vi "Actor Core.vi"(8 "error in":errorcluster, 11 "hydraharp_panel in":refnum<class "picoharp_panel.lvclass">) -> (0 "error out":errorcluster, 3 "Actor out":refnum<class "Actor.lvclass">)   [LabVIEW 2015, in "picoharp_panel.lvclass"]
doc: "(<B>Filename</B>: Actor Framework.lvlib:Actor.lvclass:Actor Core.vi)\n\nReceives messages to the actor, reacts to them, and initiates any error handling that may shut the actor down.\n\nDescendant classes may override this VI to append parallel tasks for the actor to complete while it handles messages. Overrides use the Call Parent Method node."
uses:
  picoharp_panel.lvclass
  <vilib>/ActorFramework/Actor/Actor.lvclass
  Hydraharp/hydraharp_panel/hpanel_hydraharp_settings.ctl
  Hydraharp/hydraharp_panel/hpanel_sync_settings.ctl
  Hydraharp/hydraharp_panel/hpanel_sync_div.ctl
  Hydraharp/hydraharp_panel/hpanel_channel_settings.ctl
  Hydraharp/hydraharp_panel/hpanel_acq_modes.ctl
  Hydraharp/hydraharp_panel/hpanel_hydrharp_tasks.ctl
  Hydraharp/hydraharp/hydraharp_correlation_lag_settings.ctl
  Hydraharp/hydraharp/hydraharp_time_decades.ctl
  Hydraharp/hydraharp_panel/hpanel_control_references.ctl
  UI/panel_class/panel.lvclass/panel.ctl
  <vilib>/ActorFramework/Actor/Actor.lvclass/Actor.ctl
  <vilib>/ActorFramework/Message Enqueuer/Message Enqueuer.lvclass/Message Enqueuer.ctl
  picoharp_panel.lvclass/picoharp_panel.ctl
  picoharp_panel Messages/ppanel_connect_to_hydraharp Msg/ppanel_connect_to_hydraharp Msg.lvclass/ppanel_connect_to_hydraharp Msg.ctl
  record_type.ctl
  Hydraharp/hydraharp/hydraharp_action_on_records.ctl
  picoharp_panel Messages/ppanel_stream_TTTR Msg/ppanel_stream_TTTR Msg.lvclass/ppanel_stream_TTTR Msg.ctl
  Hydraharp/hydraharp_panel/hpanel_correlation_settings.ctl
  picoharp_panel Messages/ppanel_change_hydraharp_settings Msg/ppanel_change_hydraharp_settings Msg.lvclass/ppanel_change_hydraharp_settings Msg.ctl
  <vilib>/ActorFramework/Message Enqueuer/Init from Existing Queue.vi
  <vilib>/ActorFramework/Message Enqueuer/Enqueue.vi
  <vilib>/ActorFramework/Message Priority Queue/Priority Enqueue.vi
  <vilib>/ActorFramework/Message Enqueuer/Message Enqueuer.lvclass
  picoharp_panel Messages/ppanel_disconnect_from_hydraharp Msg/ppanel_disconnect_from_hydraharp Msg.lvclass
  picoharp_panel Messages/ppanel_connect_to_hydraharp Msg/ppanel_connect_to_hydraharp Msg.lvclass
  picoharp_panel Messages/ppanel_get_current_count_rates Msg/ppanel_get_current_count_rates Msg.lvclass
  picoharp_panel Messages/ppanel_stream_TTTR Msg/ppanel_stream_TTTR Msg.lvclass
  picoharp_panel Messages/ppanel_change_hydraharp_settings Msg/ppanel_change_hydraharp_settings Msg.lvclass
  UI/panel_class/panel.lvclass
panel:
  in  "stop_task":bool
  in  "do_task":bool
  in  "Task":T1
  in  "chart_channels":bool
  in  "Mode":T2=2 items=["T2"=2, "T3"=3]
  out "Status":string
  in  "connect_hydraharp":bool
  in  "hydra_tab":enum32{"Basic Settings", "Advanced"}(tab)
  in  "Hydraharp Settings":T3={"Sync Settings"={"snc_count"=0, "snc_level"=50, "snc_ZeroX"=10, "snc_offs"=0, "sync_div"=enum."1"}, "CH 1"={"ch_counts"=0, "ch_level"=270, "ch_ZeroX"=10, "ch_offs"=0}, "CH 2"={"ch_counts"=0, "ch_level"=680, "ch_ZeroX"=10, "ch_offs"=0}, "CH 3"={"ch_counts"=0, "ch_level"=50, "ch_ZeroX"=10, "ch_offs"=0}, "CH 4"={"ch_counts"=0, "ch_level"=50, "ch_ZeroX"=10, "ch_offs"=0}, "binning"=1, "CH 5"={"ch_counts"=0, "ch_level"=0, "ch_ZeroX"=0, "ch_offs"=0}, "CH 6"={"ch_counts"=0, "ch_level"=0, "ch_ZeroX"=0, "ch_offs"=0}, "CH 7"={"ch_counts"=0, "ch_level"=0, "ch_ZeroX"=0, "ch_offs"=0}, "CH 8"={"ch_counts"=0, "ch_level"=0, "ch_ZeroX"=0, "ch_offs"=0}} {"CH 8"."ch_offs" min=-99999 max=99999 step=1; "CH 8"."ch_ZeroX" min=0 max=20 step=1; "CH 8"."ch_level" min=0 max=800 step=1; "CH 7"."ch_offs" min=-99999 max=99999 step=1; "CH 7"."ch_ZeroX" min=0 max=20 step=1; "CH 7"."ch_level" min=0 max=800 step=1; "CH 6"."ch_offs" min=-99999 max=99999 step=1; "CH 6"."ch_ZeroX" min=0 max=20 step=1; "CH 6"."ch_level" min=0 max=800 step=1; "CH 5"."ch_offs" min=-99999 max=99999 step=1; "CH 5"."ch_ZeroX" min=0 max=20 step=1; "CH 5"."ch_level" min=0 max=800 step=1; "binning" min=0 max=10 step=1; "CH 4"."ch_offs" min=-99999 max=99999 step=1; "CH 4"."ch_ZeroX" min=0 max=20 step=1; "CH 4"."ch_level" min=0 max=800 step=1; "CH 3"."ch_offs" min=-99999 max=99999 step=1; "CH 3"."ch_ZeroX" min=0 max=20 step=1; "CH 3"."ch_level" min=0 max=800 step=1; "CH 2"."ch_offs" min=-99999 max=99999 step=1; "CH 2"."ch_ZeroX" min=0 max=20 step=1; "CH 2"."ch_level" min=0 max=800 step=1; "CH 1"."ch_offs" min=-99999 max=99999 step=1; "CH 1"."ch_ZeroX" min=0 max=20 step=1; "CH 1"."ch_level" min=0 max=800 step=1; "Sync Settings"."snc_offs" min=-99999 max=99999 step=1; "Sync Settings"."snc_ZeroX" min=0 max=20 step=1; "Sync Settings"."snc_level" min=0 max=800 step=10}
  in  "acq_time (s)":u32=100
  in  "Stream Path":path
  in  "Ch2":u8 max=16
  in  "Ch1":u8 max=16
  in  "Lag Settings":T7={"time_start"=1000000, "time_end"=100000000000, "coarseness"=4} {"time_start" items=["1 ps"=1, "10 ps"=10, "100 ps"=100, "1 ns"=1000, "10 ns"=10000, "100 ns"=100000, "1 us"=1000000, "10 us"=10000000, "100 us"=100000000, "1 ms"=1000000000, "10 ms"=10000000000, "100 ms"=100000000000, "1 s"=1000000000000, "10 s"=10000000000000, "100 s"=100000000000000]; "time_end" items=["1 ps"=1, "10 ps"=10, "100 ps"=100, "1 ns"=1000, "10 ns"=10000, "100 ns"=100000, "1 us"=1000000, "10 us"=10000000, "100 us"=100000000, "1 ms"=1000000000, "10 ms"=10000000000, "100 ms"=100000000000, "1 s"=1000000000000, "10 s"=10000000000000, "100 s"=100000000000000]}
  in  "Save Records?":bool
  # "PicoHarp"
  # "CH 0"
  # "CH 1"
  # "Stream Settings"
  # "Correlation Settings"
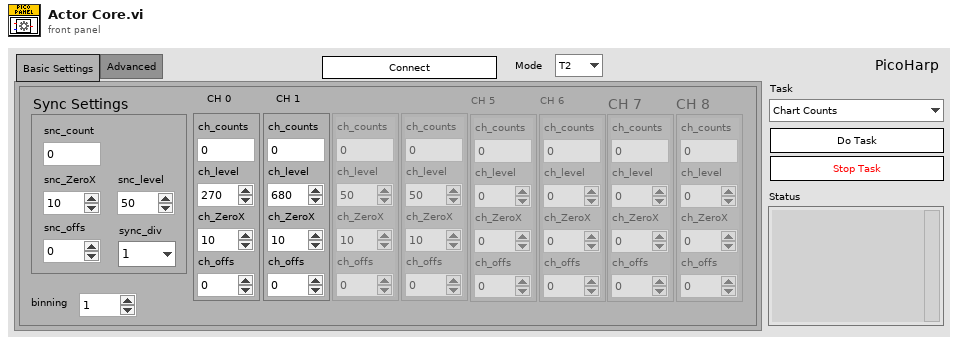
[diagram p1: front panel]
types:
  T1 = typedef "hpanel_hydrharp_tasks.ctl" = enum16{"Chart Counts", "Stream to File", "Plot Correlation"}
  T2 = typedef "hpanel_acq_modes.ctl" = u16
  T3 = typedef "hpanel_hydraharp_settings.ctl" = cluster{"Sync Settings":T4, "CH 1":T6, "CH 2":T6, "CH 3":T6, "CH 4":T6, "binning":i32, "CH 5":T6, "CH 6":T6, "CH 7":T6, "CH 8":T6}
  T4 = typedef "hpanel_sync_settings.ctl" = cluster{"snc_count":i32, "snc_level":i32, "snc_ZeroX":i32, "snc_offs":i32, "sync_div":T5}
  T5 = typedef "hpanel_sync_div.ctl" = enum16{"1", "2", "4", "8"}
  T6 = typedef "hpanel_channel_settings.ctl" = cluster{"ch_counts":i32, "ch_level":i32, "ch_ZeroX":i32, "ch_offs":i32}
  T7 = typedef "hydraharp_correlation_lag_settings.ctl" = cluster{"time_start":T8, "time_end":T8, "coarseness":i64}
  T8 = typedef "hydraharp_time_decades.ctl" = i64
  T9 = typedef "hpanel_control_references.ctl" = cluster{"Status":refnum<vi>, "snc_count":refnum<vi>, "ch1_counts":refnum<vi>, "ch2_counts":refnum<vi>, "ch3_counts":refnum<vi>, "ch4_counts":refnum<vi>, "ch5_counts":refnum<vi>, "ch6_counts":refnum<vi>, "ch7_counts":refnum<vi>, "ch8_counts":refnum<vi>}
  T10 = typedef "hpanel_user_events.ctl" = cluster{"message_panel":refnum<event-registration>, "stop_fifo_stream":refnum<event-registration>, "harp_status":refnum<event-registration>}
  T11 = cluster{"message_panel":refnum<event-registration>, "stop_ui_ref":refnum<event-registration>, "harp_status":refnum<event-registration>}
  T12 = typedef "record_type.ctl" = enum16{"Raw Stream", "Processed Records (hdf5)"}
  T13 = enum8{"Enabled", "Disabled", "Disabled and Grayed Out"}
  T14 = typedef "hydraharp_action_on_records.ctl" = enum16{"stream_to_file", "correlate", "stream to file and correlate"}
  T15 = typedef "hpanel_correlation_settings.ctl" = cluster{"Lag Settings":T7, "Ch1":u8, "Ch2":u8}
  T16 = typedef "ui_user_events.ctl" = cluster{"update_xy_graph":refnum<user-event>, "update_graph":refnum<user-event>, "update_chart":refnum<user-event>, "update_map":refnum<user-event>, "event_loop_stop":refnum<user-event>, "keep_map":refnum<user-event>}
  T17 = typedef "hydrharp_tasks.ctl" = enum16{"Chart Counts", "Stream to File", "Plot Correlation"}
  T18 = typedef "messages_to_panel_from_actor_loop.ctl" = enum16{"reenable_tasks"}
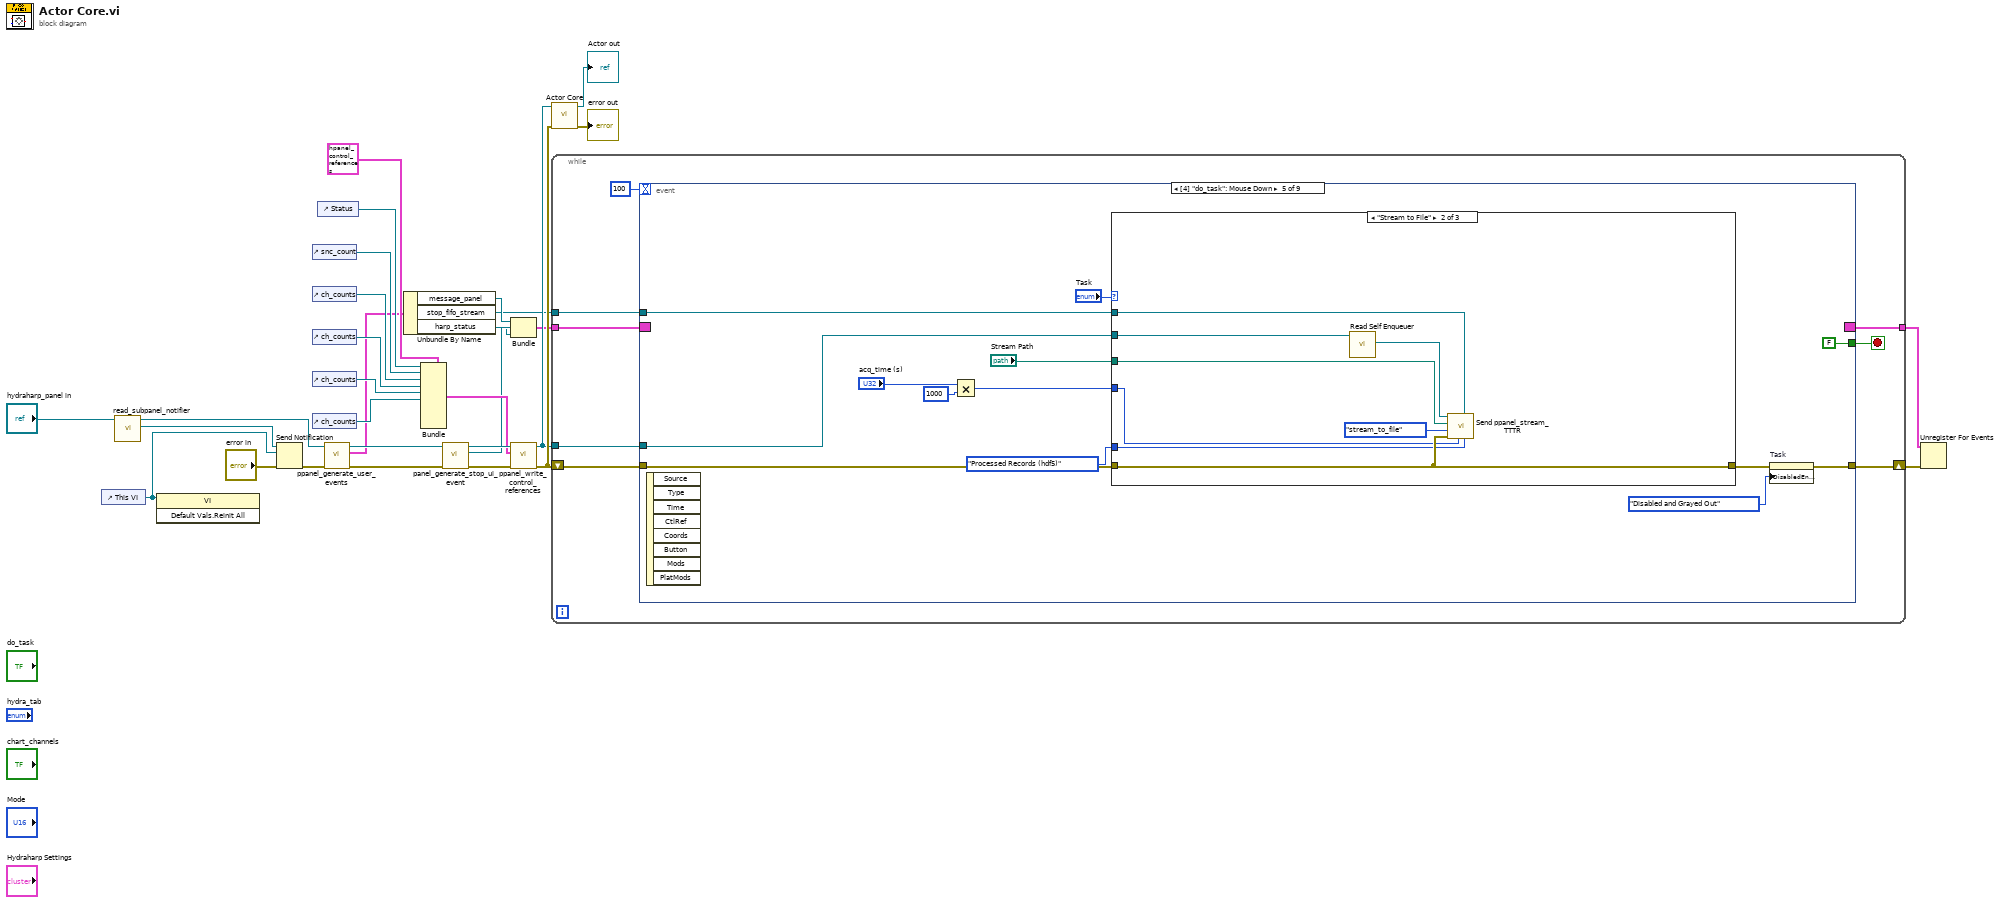
[diagram p0: block diagram]
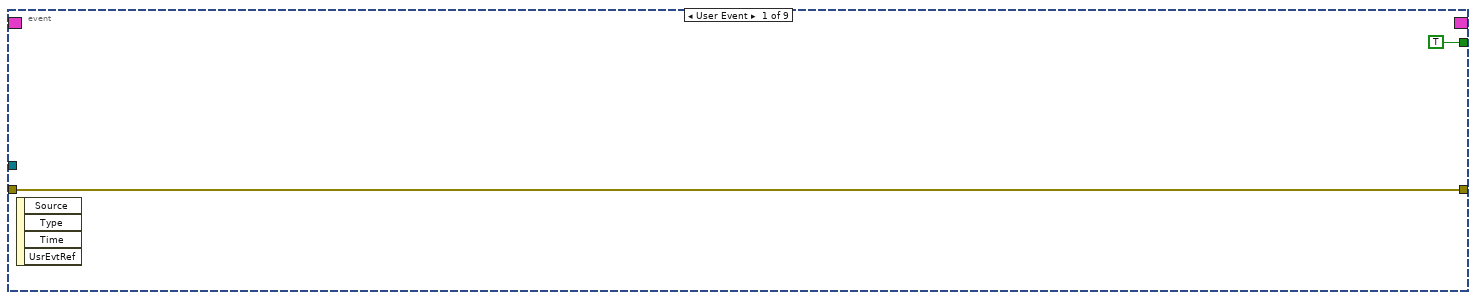
[diagram p2: hidden frame]
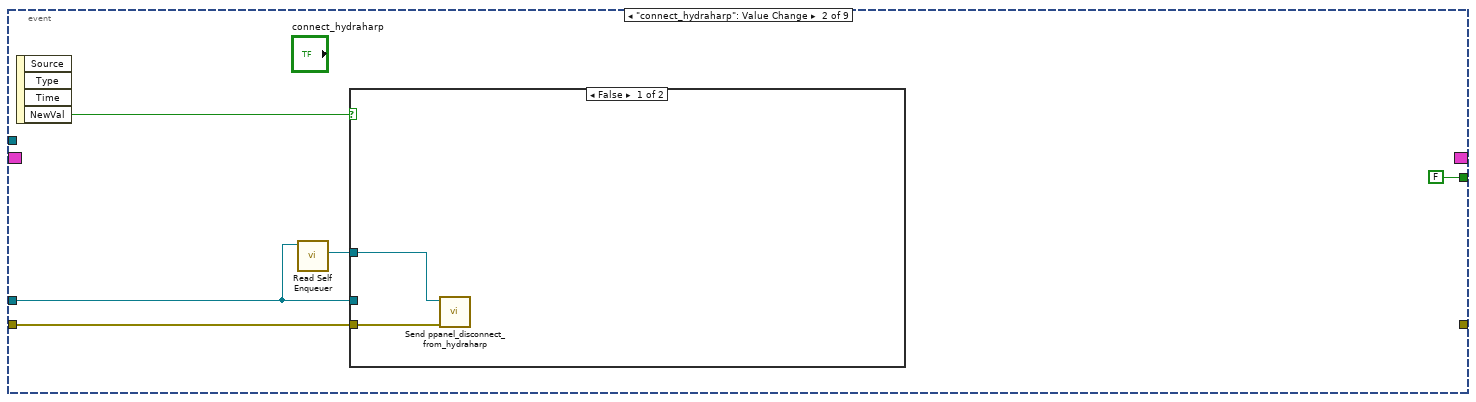
[diagram p3: hidden frame]
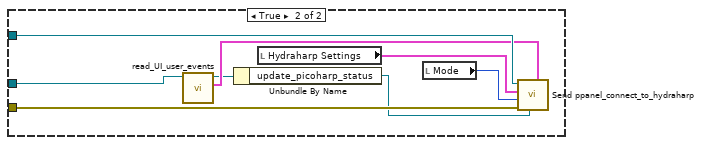
[diagram p4: hidden frame]
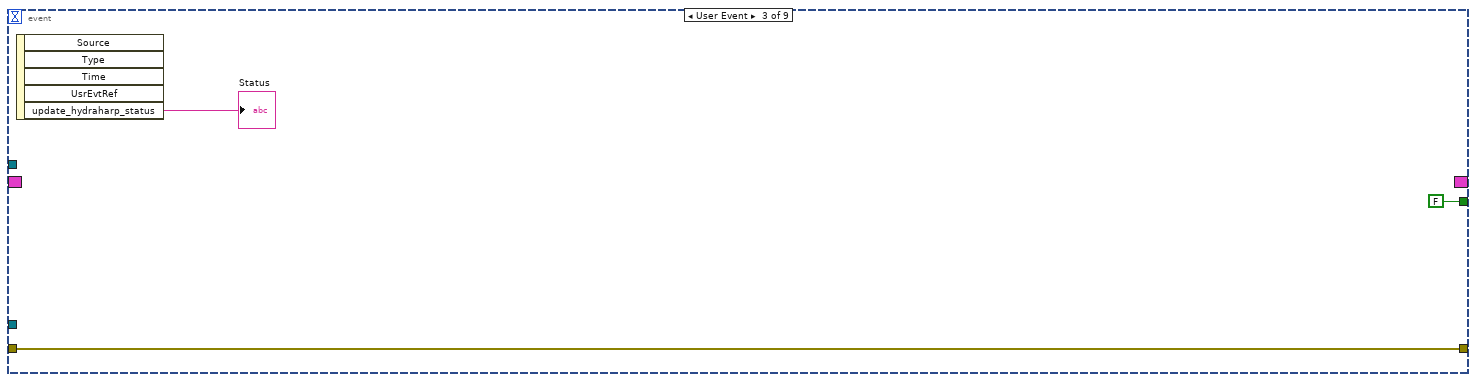
[diagram p5: hidden frame]
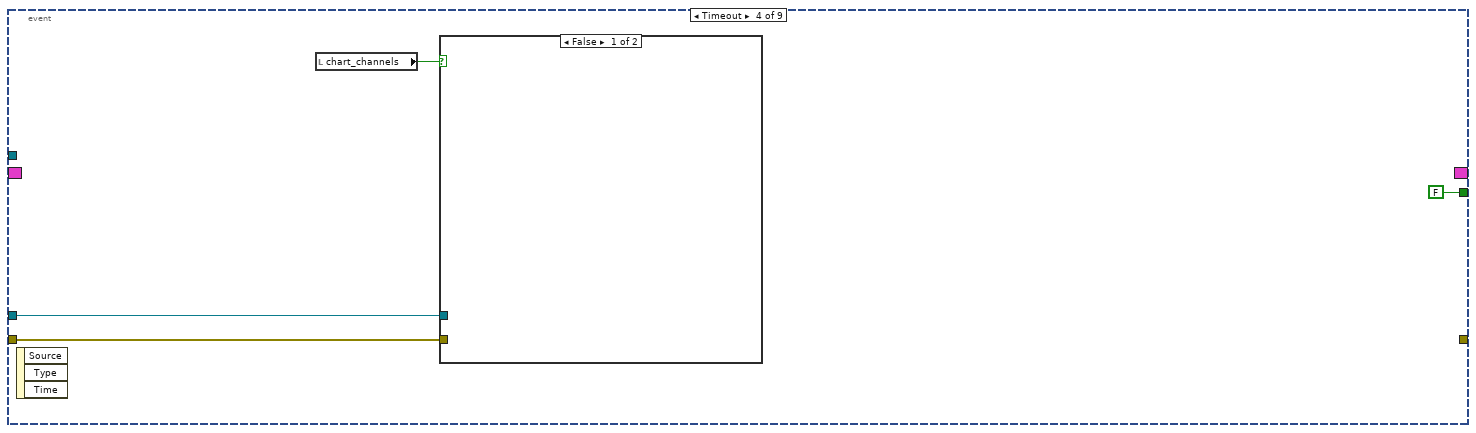
[diagram p6: hidden frame]
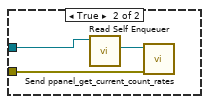
[diagram p7: hidden frame]
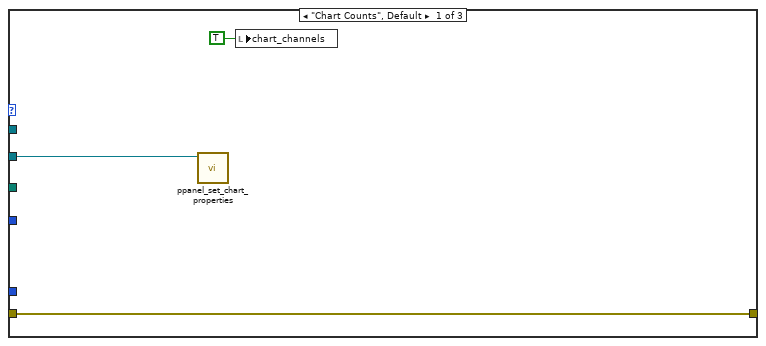
[diagram p8: hidden frame]
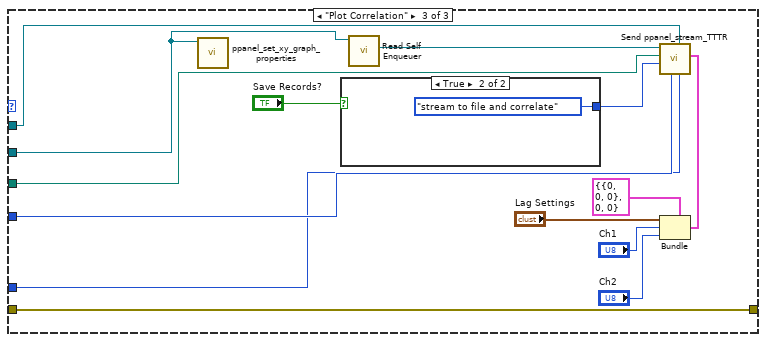
[diagram p9: hidden frame]
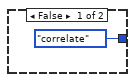
[diagram p10: hidden frame]
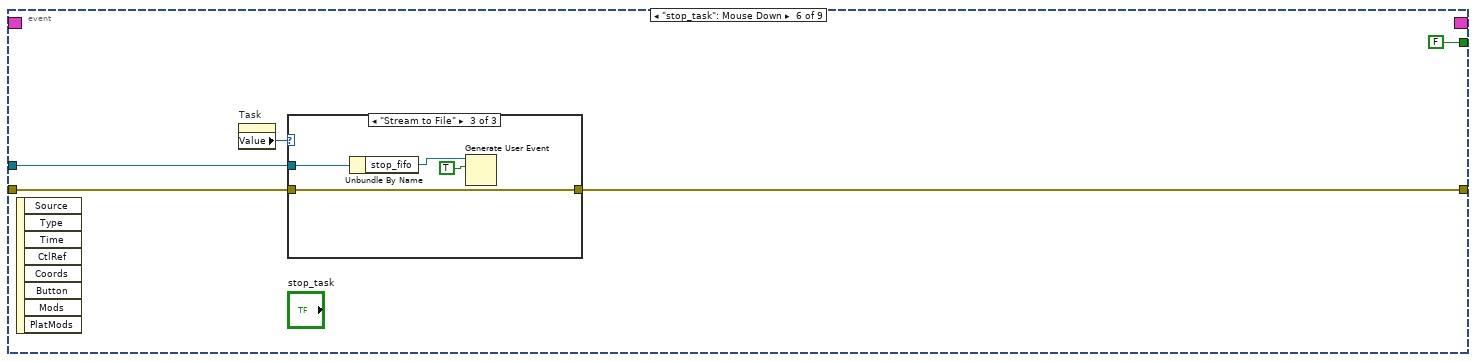
[diagram p11: hidden frame]
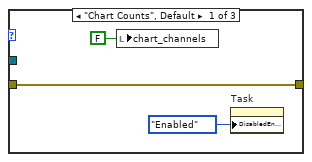
[diagram p12: hidden frame]
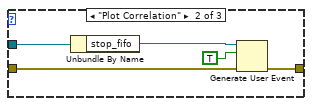
[diagram p13: hidden frame]
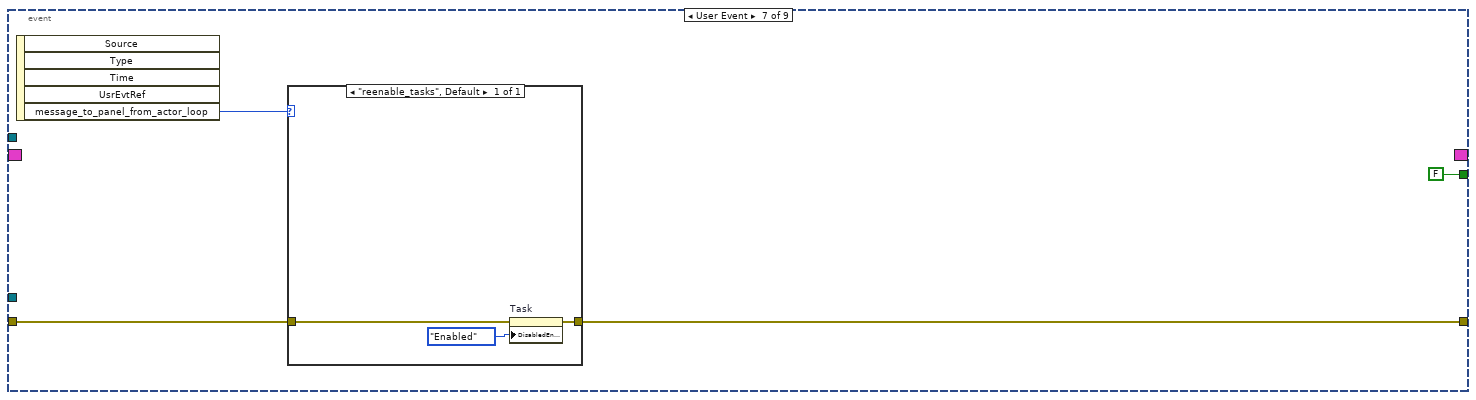
[diagram p14: hidden frame]
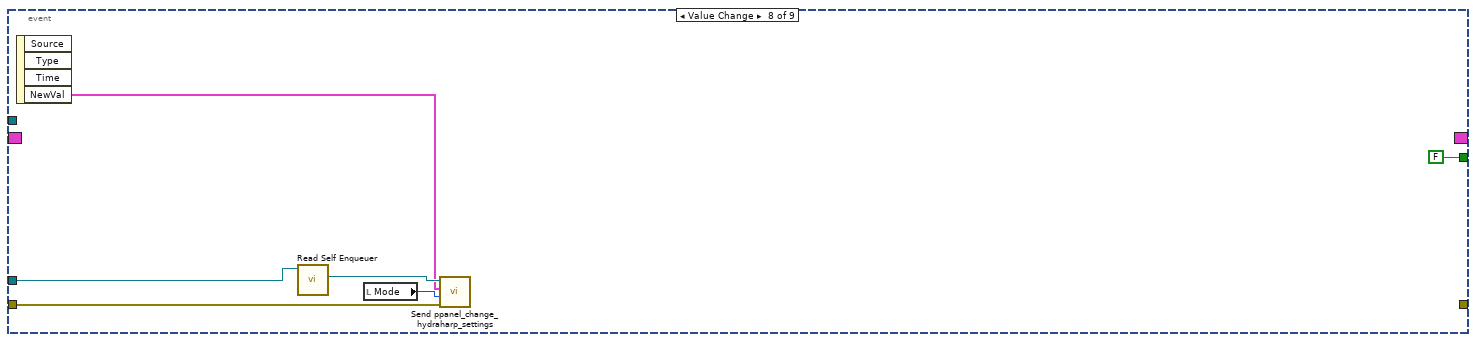
[diagram p15: hidden frame]
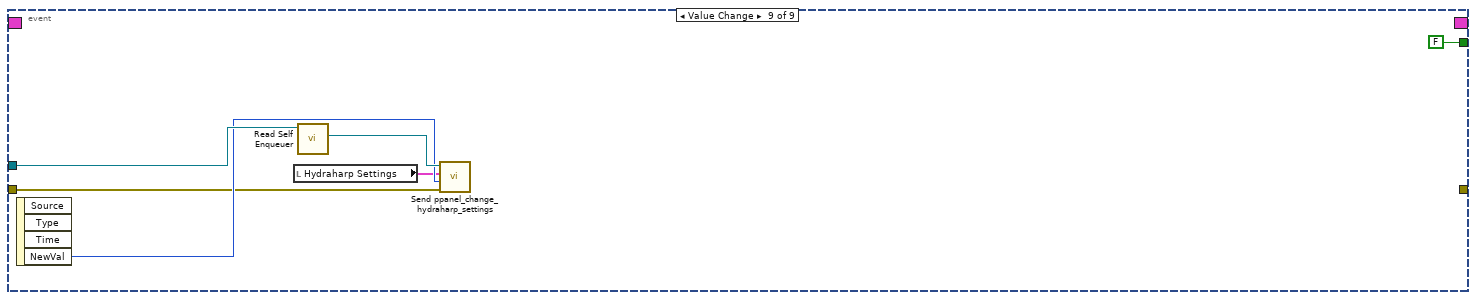
[diagram p16: hidden frame]
diagram:
  n1 = control-ref of="This VI"() -> (w13:refnum<vi>)
  n2 = call "read_subpanel_notifier.vi"("panel in"="hydraharp_panel in") -> ("subpanel_notifier"=w1:refnum<notifier>, "panel out"=w2:refnum<class "picoharp_panel.lvclass">)  [unwired: 8 in, 1 out]
  n3 = invoke class="VI" method="Default Vals.Reinit All"(reference=w13) -> ()  [unwired: 2 in, 3 out]
  n4 = Send Notification(notification=w13, notifier=w1, error in (no error)="error in") -> (error out=w12:errorcluster)  [unwired: 1 out]
  n5 = control-ref of="snc_count"() -> (w24:refnum<vi>)
  n6 = control-ref of="ch_counts"() -> (w23:refnum<vi>)
  n7 = control-ref of="ch_counts"() -> (w22:refnum<vi>)
  n8 = control-ref of="ch_counts"() -> (w21:refnum<vi>)
  n9 = control-ref of="ch_counts"() -> (w20:refnum<vi>)
  n10 = control-ref of="Status"() -> (w25:refnum<vi>)
  n11 = call "ppanel_generate_user_events.vi"("error in (no error)"=w12, "picoharp_panel in"=w2) -> ("error out"=w11:errorcluster, "events"=w8:T10, "hydraharp_panel out"=w10:refnum<class "picoharp_panel.lvclass">)  [unwired: 7 in]
  n12 = Unbundle By Name(w8) -> ("message_panel"=w7:refnum<event-registration>, "stop_fifo_stream"=w5:refnum<event-registration>, "harp_status"=w4:refnum<event-registration>)
  n13 = Bundle(cluster=T9 {"Status"=refnum, "snc_count"=refnum, "ch1_counts"=refnum, "ch2_counts"=refnum, "ch3_counts"=refnum, "ch4_counts"=refnum, "ch5_counts"=refnum, "ch6_counts"=refnum, "ch7_counts"=refnum, "ch8_counts"=refnum} ("output cluster"), "Status"=w25, "snc_count"=w24, "ch1_counts"=w23, "ch2_counts"=w22, "ch3_counts"=w21, "ch4_counts"=w20) -> (w15:T9)  [unwired: 4 in]
  n14 = call "panel_generate_stop_ui_event.vi"("error in (no error)"=w11, "panel in"=w10) -> ("error out"=w17:errorcluster, "stop_ui_ref"=w9:refnum<event-registration>, "panel out"=w18:refnum<class "picoharp_panel.lvclass">)  [unwired: 7 in]
  n15 = Bundle("message_panel"=w7, "stop_ui_ref"=w9, "harp_status"=w4) -> (w6:T11)  [unwired: 1 in]
  n16 = call "ppanel_write_control_references.vi"("error in (no error)"=w17, "references"=w15, "hydraharp_panel in"=w18) -> ("error out"=w16:errorcluster, "hydraharp_panel out"=w14:refnum<class "picoharp_panel.lvclass">)  [unwired: 7 in]
  n17 = call-parent "Actor Core.vi"("error in"=w16, "Actor in"=w14) -> ("error out"=→"error out":errorcluster, "Actor out"=→"Actor out":refnum<class "Actor.lvclass">)  [unwired: 8 in]
  n18 = while {
    tunnel: [w38] -> w27
    shift-right: [w35] -> w26
    shift-left: w16 -> [w36]
    tunnel: w14 -> [w34]
    tunnel: w6 -> [w32]
    tunnel: w5 -> [w31]
    stop <- w37 stop-if-true
    n19 = event shown="[4] \"do_task\": Mouse Down" {
      selector: w32 -> [_ _ _ _ _ _ _ _ _]
      dyn-events: [_ _ _ _ _ _ _ _ _] -> w38
      timeout: 100 -> [_ _ _ _ _ _ _ _ _]
      tunnel: [TRUE FALSE FALSE FALSE FALSE FALSE FALSE FALSE FALSE] -> w37
      tunnel: w36 -> [w39 w45 w56 w60 w76 w109 w124 w130 w137]
      tunnel: [w39 _ w56 _ w74 w106 w123 _ _] -> w35
      tunnel: w34 -> [_ w41 _ w61 w72 w107 _ w135 w141]
      tunnel: w31 -> [_ _ _ _ w71 _ _ _ _]
      event User Event {
        n20 = event-data() -> ()  [unwired: 1 in, 4 out]
      }
      event "connect_hydraharp": Value Change {
        n21 = event-data() -> ("NewVal"=w43:bool)  [unwired: 1 in, 3 out]
        n22 = call <vilib>:"Read Self Enqueuer.vi"("Actor"=w41) -> ("Self Enqueuer"=w44:refnum<class "Message Enqueuer.lvclass">)  [unwired: 10 in]
        n23 = case shown="False" w43 {
          tunnel: w45 -> [w46 w55]
          tunnel: w44 -> [w47 w54]
          tunnel: w41 -> [_ w50]
          frame False {
            n24 = call "Send ppanel_disconnect_from_hydraharp.vi"("error in (no error)"=w46, "Message Enqueuer"=w47) -> ()  [unwired: 8 in, 2 out]
          }
          frame True {
            n25 = call "read_UI_user_events.vi"("panel in"=w50) -> ("ui_user_events"=w49:T16, "panel out"=w48:refnum<class "picoharp_panel.lvclass">)  [unwired: 8 in, 1 out]
            n26 = Unbundle By Name(w48) -> ("update_picoharp_status"=w51:refnum<user-event>)
            n27 = local read "Hydraharp Settings"() -> (w53:T3)
            n28 = local read "Mode"() -> (w52:T2)
            n29 = call "Send ppanel_connect_to_hydraharp.vi"("ui_events"=w49, "update_hydraharp_status"=w51, "error in (no error)"=w55, "Mode"=w52, "Hydraharp Settings"=w53, "Message Enqueuer"=w54) -> ()  [unwired: 4 in, 2 out]
          }
        }
      }
      event User Event {
        n30 = event-data() -> ("update_hydraharp_status"=→"Status":string)  [unwired: 1 in, 4 out]
      }
      event Timeout {
        n31 = event-data() -> ()  [unwired: 1 in, 3 out]
        n32 = local read "chart_channels"() -> (w59:bool)
        n33 = case shown="False" w59 {
          tunnel: w61 -> [_ w65]
          tunnel: w60 -> [_ w63]
          frame False {
          }
          frame True {
            n34 = call <vilib>:"Read Self Enqueuer.vi"("Actor"=w65) -> ("Self Enqueuer"=w64:refnum<class "Message Enqueuer.lvclass">)  [unwired: 10 in]
            n35 = call "Send ppanel_get_current_count_rates.vi"("error in (no error)"=w63, "Message Enqueuer"=w64) -> ()  [unwired: 8 in, 2 out]
          }
        }
      }
      event "do_task": Mouse Down {
        n36 = event-data() -> ()  [unwired: 1 in, 8 out]
        n37 = Multiply(x="acq_time (s)", y=u32 1000) -> (x*y=w67:u32)
        n38 = case shown="\"Stream to File\"" "Task" {
          tunnel: w76 -> [w81 w89 w94]
          tunnel: [w81 w89 w94] -> w75
          tunnel: w72 -> [w79 w83 w92]
          tunnel: w71 -> [_ w86 w91]
          tunnel: "Stream Path" -> [_ w85 w97]
          tunnel: record_type."Processed Records (hdf5)" ("Record Type") -> [_ w82 w90]
          tunnel: w67 -> [_ w84 w96]
          frame "Chart Counts", Default {
            n39 = call "ppanel_set_chart_properties.vi"("hydraharp_panel in"=w79) -> ()  [unwired: 11 in]
            n40 = local write "chart_channels"(TRUE ("chart_channels")) -> ()
          }
          frame "Stream to File" {
            n41 = call <vilib>:"Read Self Enqueuer.vi"("Actor"=w83) -> ("Self Enqueuer"=w88:refnum<class "Message Enqueuer.lvclass">)  [unwired: 10 in]
            n42 = call "Send ppanel_stream_TTTR.vi"("Record Type"=w82, "stop_fifo_event"=w86, "acq_time"=w84, "error in (no error)"=w89, "action_for_records"=hydraharp_action_on_records."stream_to_file", "fifo_stream_path"=w85, "Message Enqueuer"=w88) -> ()  [unwired: 3 in, 2 out]
          }
          frame "Plot Correlation" {
            n43 = call "ppanel_set_xy_graph_properties.vi"("hydraharp_panel in"=w92) -> ()  [unwired: 11 in]
            n44 = case shown="True" "Save Records?" {
              tunnel: [hydraharp_action_on_records."correlate" ("action_for_records") hydraharp_action_on_records."stream to file and correlate" ("action_for_records")] -> w95
              frame False {
              }
              frame True {
              }
            }
            n45 = call <vilib>:"Read Self Enqueuer.vi"("Actor"=w92) -> ("Self Enqueuer"=w98:refnum<class "Message Enqueuer.lvclass">)  [unwired: 10 in]
            n46 = Bundle(cluster=T15 {"Lag Settings"={"time_start"=0, "time_end"=0, "coarseness"=0}, "Ch1"=0, "Ch2"=0} ("output cluster"), "Lag Settings"="Lag Settings", "Ch1"="Ch1", "Ch2"="Ch2") -> (w99:T15)
            n47 = call "Send ppanel_stream_TTTR.vi"("Correlation_settings"=w99, "Record Type"=w90, "stop_fifo_event"=w91, "acq_time"=w96, "action_for_records"=w95, "fifo_stream_path"=w97, "Message Enqueuer"=w98) -> ()  [unwired: 3 in, 2 out]
          }
        }
        n48 = property on="Task" class="Enum (strict)"(error in=w75, "DisabledEnum"=T13."Disabled and Grayed Out" ("Disabled")) -> (error out=w74:errorcluster)  [unwired: 1 in, 1 out]
      }
      event "stop_task": Mouse Down {
        n49 = event-data() -> ()  [unwired: 1 in, 8 out]
        n50 = property on="Task" class="Enum (strict)"() -> ("Value"=w110:T17)  [unwired: 2 in, 2 out]
        n51 = case shown="\"Stream to File\"" w110 {
          tunnel: w109 -> [w112 w115 w121]
          tunnel: [w112 w114 w121] -> w106
          tunnel: w107 -> [_ w116 w120]
          frame "Chart Counts", Default {
            n52 = local write "chart_channels"(FALSE ("chart_channels")) -> ()
            n53 = property on="Task" class="Enum (strict)"("DisabledEnum"=T13."Enabled" ("Disabled")) -> ()  [unwired: 2 in, 2 out]
          }
          frame "Plot Correlation" {
            n54 = Unbundle By Name(w116) -> ("stop_fifo"=w117:refnum<user-event>)
            n55 = Generate User Event(user event=w117, event data cluster=TRUE ("event data"), error in=w115) -> (error out=w114:errorcluster)  [unwired: 1 in, 1 out]
          }
          frame "Stream to File" {
            n56 = Unbundle By Name(w120) -> ("stop_fifo"=w119:refnum<user-event>)
            n57 = Generate User Event(user event=w119, event data cluster=TRUE ("event data")) -> ()  [unwired: 2 in, 2 out]
          }
        }
      }
      event User Event {
        n58 = event-data() -> ("message_to_panel_from_actor_loop"=w126:T18)  [unwired: 1 in, 4 out]
        n59 = case shown="\"reenable_tasks\", Default" w126 {
          tunnel: w124 -> [w128]
          tunnel: [w127] -> w123
          frame "reenable_tasks", Default {
            n60 = property on="Task" class="Enum (strict)"(error in=w128, "DisabledEnum"=T13."Enabled" ("Disabled")) -> (error out=w127:errorcluster)  [unwired: 1 in, 1 out]
          }
        }
      }
      event Value Change {
        n61 = event-data() -> ("NewVal"=w133:T3)  [unwired: 1 in, 3 out]
        n62 = call <vilib>:"Read Self Enqueuer.vi"("Actor"=w135) -> ("Self Enqueuer"=w134:refnum<class "Message Enqueuer.lvclass">)  [unwired: 10 in]
        n63 = local read "Mode"() -> (w132:T2)
        n64 = call "Send ppanel_change_hydraharp_settings.vi"("error in (no error)"=w130, "Mode"=w132, "Hydraharp Settings"=w133, "Message Enqueuer"=w134) -> ()  [unwired: 6 in, 2 out]
      }
      event Value Change {
        n65 = event-data() -> ("NewVal"=w139:T2)  [unwired: 1 in, 3 out]
        n66 = local read "Hydraharp Settings"() -> (w138:T3)
        n67 = call <vilib>:"Read Self Enqueuer.vi"("Actor"=w141) -> ("Self Enqueuer"=w140:refnum<class "Message Enqueuer.lvclass">)  [unwired: 10 in]
        n68 = call "Send ppanel_change_hydraharp_settings.vi"("error in (no error)"=w137, "Mode"=w139, "Hydraharp Settings"=w138, "Message Enqueuer"=w140) -> ()  [unwired: 6 in, 2 out]
      }
    }
  }
  n69 = Unregister For Events(event registration refnum=w27, error in=w26) -> ()  [unwired: 1 out]
